vi "Query with Scalar Double Result.vi"(8 "error in (no error)":errorcluster, 10 "Query string":string, 11 "sqlite3 in":refnum<class "sqlite3.lvclass">) -> (0 "error out":errorcluster, 2 "Result":dbl, 3 "sqlite3 out":refnum<class "sqlite3.lvclass">)   [LabVIEW 2020, in "sqlite3.lvlib" / "sqlite3.lvclass"]
uses:
  sqlite3.lvclass
  sqlite3.lvclass/sqlite3.ctl
  714d8927-150b-4709-a607-ab2129c733ff.vi
  sqlite/VIs/open v2.vi
  sqlite/VIs/close v2.vi
  sqlite/VIs/prepare v2.vi
  sqlite/VIs/step.vi
  sqlite/VIs/column count.vi
  db layer/compound/Resolve Result Type.vi
  714d8927-150b-4709-a607-ab2129c733ff.vi/0244caef-bc9a-4150-a8ac-bf3d364b181c.vi
  714d8927-150b-4709-a607-ab2129c733ff.vi/5568208c-18c9-421a-afbc-e39208249946.vi
  sqlite/VIs/finalize.vi
  sqlite/subvi/Error Converter (ErrCode or Status).vi
  sqlite/VIs/column type.vi
  sqlite/VIs/column double.vi
  714d8927-150b-4709-a607-ab2129c733ff.vi/0244caef-bc9a-4150-a8ac-bf3d364b181c.vi/a2f834d3-bc69-4783-ae95-d707ddaccc14.vi
  714d8927-150b-4709-a607-ab2129c733ff.vi/5568208c-18c9-421a-afbc-e39208249946.vi/01062d92-5897-4021-bc82-797811f63e93.vi
  sqlite/VIs/errstr.vi
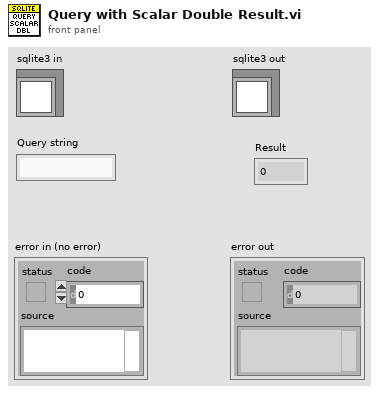
[diagram p1: front panel]
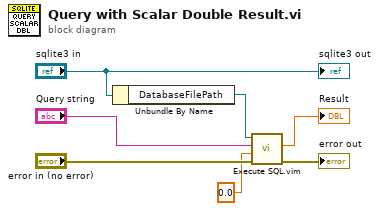
[diagram p0: block diagram]
diagram:
  n1 = Unbundle By Name("sqlite3 in") -> ("DatabaseFilePath"=w7:path)
  n2 = call "Execute SQL.vim"("error in (no error)"="error in (no error)", "desired return type(none)"=0.0, "sql (string)"="Query string", "database in"=w7) -> ("error out"=→"error out":errorcluster, "Query Result"=→"Result":dbl)  [unwired: 6 in]
  "sqlite3 out" <- "sqlite3 in"
